vi "XY Graph Set TipStrip Visible.vi"(8 "error in (no error)":errorcluster, 10 "TipStrip Visible":bool, 11 "XY Graph Refnum":T1) -> (0 "error out":errorcluster, 2 "TipStrip Refnum":refnum<vi>, 3 "XY Graph Refnum (dup)":T1)   [LabVIEW 2021, in "XY Graph Add-Ons.lvlib"]
uses:
  XY Graph Add-Ons.lvlib
  XY Graph Refnum.ctl
  XY Graph Property Tag List.ctl
  7791d90f-93c4-456f-91dc-950c551374c4.vi
  <vilib>/UserTags/UserTags.lvlib
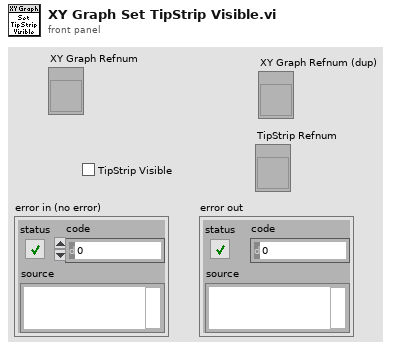
[diagram p1: front panel]
types:
  T1 = typedef "XY Graph Add-Ons.lvlib/XY Graph Refnum.ctl" = refnum<vi>
  T2 = typedef "XY Graph Add-Ons.lvlib/XY Graph Property Tag List.ctl" = enum16{"Max Legend Size", "Preserved Plots", "XScales.GridColors", "YScales.GridColors", "TipStrip String", "TipStrip Visible", "Tool Panels Visibility", "Plots Metadata"}
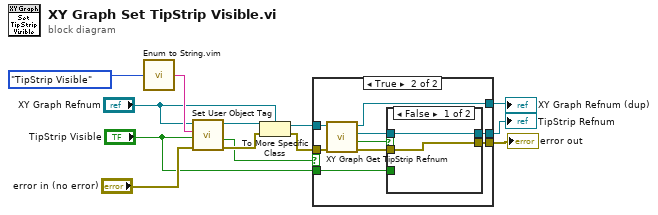
[diagram p0: block diagram]
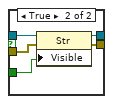
[diagram p3: hidden frame]
diagram:
  n1 = call "Enum to String.vim"("Enum"=XY_Graph_Property_Tag_List."TipStrip Visible" ("XY Graph Property Tag")) -> ("String"=w12:string)
  n2 = call <vilib>:"Set User Object Tag.vi"("error in (no error)"="error in (no error)", "Value"="TipStrip Visible", "Tag Name"=w12, "Generic Refnum"="XY Graph Refnum") -> ("error out"=w8:errorcluster, "Was Tag Set?"=w2:bool, "dup Generic Refnum"=w10:refnum<vi>)  [unwired: 5 in]
  n3 = To More Specific Class(target class="XY Graph Refnum", reference=w10, error in=w8) -> (specific class reference=w7:T1, error out=w6:errorcluster)
  n4 = case shown="True" w2 {
    tunnel: w7 -> [w15 w24]
    tunnel: w6 -> [w14 w23]
    tunnel: [w15 w21] -> w5
    tunnel: "TipStrip Visible" -> [_ w20]
    tunnel: [w14 w18] -> w3
    tunnel: [_ w16] -> w1
    frame False {
    }
    frame True {
      n5 = call "XY Graph Get TipStrip Refnum.vi"("Error In"=w23, "XYGraph Refnum"=w24) -> ("Error Out"=w19:errorcluster, "TipStrip Refnum Found?"=w17:bool, "TipStrip Refnum"=w22:refnum<vi>, "XYGraph Refnum"=w21:T1)  [unwired: 6 in]
      n6 = case shown="False" w17 {
        tunnel: w22 -> [w25 w31]
        tunnel: w20 -> [_ w30]
        tunnel: w19 -> [w26 w29]
        tunnel: [w26 w28] -> w18
        tunnel: [w25 w27] -> w16
        frame False {
        }
        frame True {
          n7 = property class="Str"(reference=w31, error in=w29, "Visible"=w30) -> (reference out=w27:refnum<vi>, error out=w28:errorcluster)
        }
      }
    }
  }
  "error out" <- w3
  "XY Graph Refnum (dup)" <- w5
  "TipStrip Refnum" <- w1
